vi "SeriellReadFPGA_ECD.vi"   [LabVIEW 2017]
uses:
  <vilib>/rvi/eio/common/nirviEmuTemplateMethod_errors.vi
  <vilib>/rvi/Emulation/niFpgaGetClockAttributes.vi
  <vilib>/rvi/Emulation/niFpgaSctlEmulationGetInTimedLoop.vi
  <vilib>/rvi/Emulation/niFpgaEmulationReportErrorSimple.vi
  GVglobalStopFPGA_ECD.vi
  <vilib>/rvi/DataTransferAndStorage/Container/Common/niFpgaContainerExecOnDevCompGetState.vi
  <vilib>/rvi/Emulation/niFpgaEmulationIsFPGAContextNoSignature.vi
  <vilib>/rvi/errors/niFpgaSetErrorForExecOnDevCompSimple.vi
  <vilib>/rvi/eio/common/nirviEmuReportErrorAndStop.vi
  <vilib>/rvi/DataTransferAndStorage/Container/Common/niFpgaContainerGetUniqueNameForEmu.vi
  <vilib>/rvi/FIFO/Fifo_Resource/nirvififoEmulationSetSize.vi
  <vilib>/rvi/FIFO/Fifo_Resource/nirviFifoEmulationQueueMgr.vi
  <instcachedir>/0/nirviFifoEmulationQueueMgr_E5CAEC123FF24DC58D834DCA3CDAA9B5.lvgen/nirviFifoEmulationQueueMgr_E5CAEC123FF24DC58D834DCA3CDAA9B5_002.vi
  <vilib>/rvi/FIFO/Fifo_Resource/nirvififoEmulationDetermineInputValidOut.vi
  <vilib>/rvi/FIFO/Fifo_Resource/nirvififoEmulationCreateLock.vi
  <vilib>/rvi/Emulation/niFpgaProcessEmulError.vi
  <vilib>/rvi/FIFO/Fifo_Resource/nirvififoEmulationObtainLock.vi
  <vilib>/rvi/FIFO/Fifo_Resource/nirvififoEmulationReleaseLock.vi
  <vilib>/rvi/occurrence/nirviWaitOnOccurrenceBase.vi
  <vilib>/rvi/errors/nirviReportUnexpectedCaseInternalError.vi
  <vilib>/rvi/errors/nirviReportUnexpectedCaseInternalError (U32).vi
  <vilib>/Utility/error.llb/Clear Errors.vi
  <vilib>/rvi/interface/RandomDataEmulation/niFpgaRandomDataHandleErrors.vi
  <vilib>/rvi/Emulation/niFpgaCriticalErrorInLSC.vi
  <vilib>/eio/EIOMethodNode/EIOMethodNode.xnode
  <vilib>/rvi/DataTransferAndStorage/Container/XNode/niFpgaContainer.xnode
  <vilib>/rvi/FIFO/Fifo_Resource/niFpgaFifoEmulationRefIn.vi
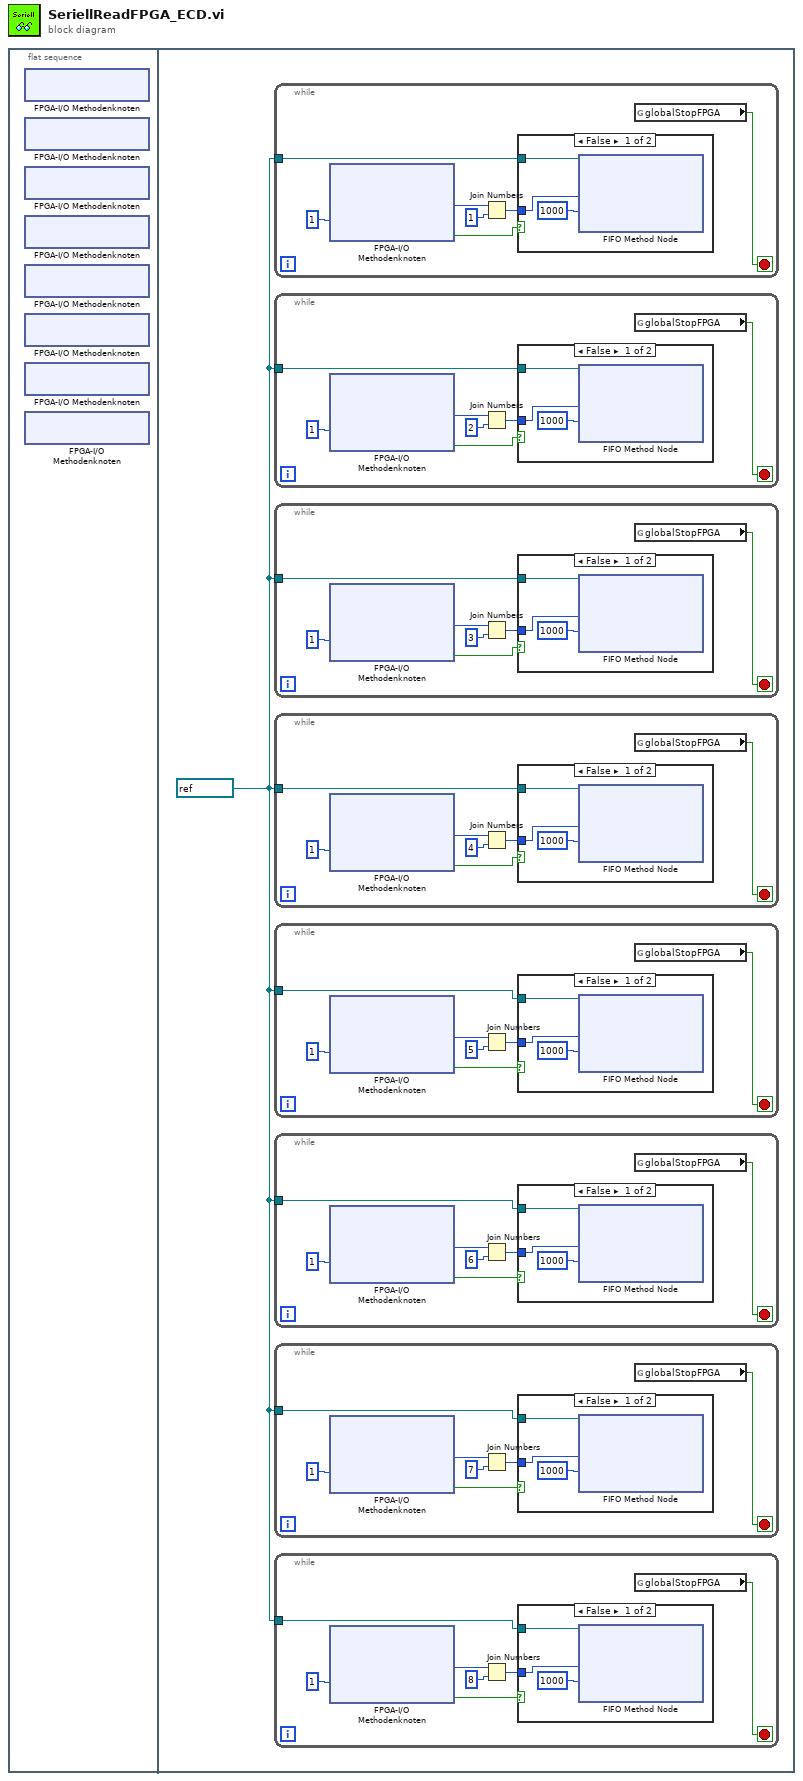
[diagram p0: block diagram]
diagram:
  n1 = flat-sequence {
    frame #0 {
      n2 = xnode "FPGA-I/O Methodenknoten"() -> ()  [unwired: 1 in, 1 out]
      n3 = xnode "FPGA-I/O Methodenknoten"() -> ()  [unwired: 1 in, 1 out]
      n4 = xnode "FPGA-I/O Methodenknoten"() -> ()  [unwired: 1 in, 1 out]
      n5 = xnode "FPGA-I/O Methodenknoten"() -> ()  [unwired: 1 in, 1 out]
      n6 = xnode "FPGA-I/O Methodenknoten"() -> ()  [unwired: 1 in, 1 out]
      n7 = xnode "FPGA-I/O Methodenknoten"() -> ()  [unwired: 1 in, 1 out]
      n8 = xnode "FPGA-I/O Methodenknoten"() -> ()  [unwired: 1 in, 1 out]
      n9 = xnode "FPGA-I/O Methodenknoten"() -> ()  [unwired: 1 in, 1 out]
    }
    frame #1 {
      w1 = refnum<k21> "READ" ("FIFO (Eingang)")
      n10 = while {
        tunnel: w1 -> [w72]
        stop <- w73 stop-if-true
        n11 = xnode "FPGA-I/O Methodenknoten"("Timeout (ms)"=1) -> ("Data"=w78:u8, "Timed Out"=w76:bool)  [unwired: 1 in, 1 out]
        n12 = Join Numbers(hi=w78, lo=u8 1) -> ((hi.lo)=w75:u16)
        n13 = case shown="False" w76 {
          tunnel: w75 -> [w81 _]
          tunnel: w72 -> [w79 _]
          frame False {
            n14 = xnode ("FIFO Method Node")("Element"=w81, "Timeout"=1000, "FIFO (Eingang)"=w79) -> ()  [unwired: 2 out]
          }
          frame True {
          }
        }
        n15 = global read "GVglobalStopFPGA_ECD.vi" "globalStopFPGA"() -> (w73:bool)
      }
      n16 = while {
        tunnel: w1 -> [w62]
        stop <- w63 stop-if-true
        n17 = xnode "FPGA-I/O Methodenknoten"("Timeout (ms)"=1) -> ("Data"=w68:u8, "Timed Out"=w66:bool)  [unwired: 1 in, 1 out]
        n18 = Join Numbers(hi=w68, lo=u8 2) -> ((hi.lo)=w65:u16)
        n19 = case shown="False" w66 {
          tunnel: w65 -> [w71 _]
          tunnel: w62 -> [w69 _]
          frame False {
            n20 = xnode ("FIFO Method Node")("Element"=w71, "Timeout"=1000, "FIFO (Eingang)"=w69) -> ()  [unwired: 2 out]
          }
          frame True {
          }
        }
        n21 = global read "GVglobalStopFPGA_ECD.vi" "globalStopFPGA"() -> (w63:bool)
      }
      n22 = while {
        tunnel: w1 -> [w52]
        stop <- w53 stop-if-true
        n23 = xnode "FPGA-I/O Methodenknoten"("Timeout (ms)"=1) -> ("Data"=w58:u8, "Timed Out"=w56:bool)  [unwired: 1 in, 1 out]
        n24 = Join Numbers(hi=w58, lo=u8 3) -> ((hi.lo)=w55:u16)
        n25 = case shown="False" w56 {
          tunnel: w55 -> [w61 _]
          tunnel: w52 -> [w59 _]
          frame False {
            n26 = xnode ("FIFO Method Node")("Element"=w61, "Timeout"=1000, "FIFO (Eingang)"=w59) -> ()  [unwired: 2 out]
          }
          frame True {
          }
        }
        n27 = global read "GVglobalStopFPGA_ECD.vi" "globalStopFPGA"() -> (w53:bool)
      }
      n28 = while {
        tunnel: w1 -> [w42]
        stop <- w43 stop-if-true
        n29 = xnode "FPGA-I/O Methodenknoten"("Timeout (ms)"=1) -> ("Data"=w48:u8, "Timed Out"=w46:bool)  [unwired: 1 in, 1 out]
        n30 = Join Numbers(hi=w48, lo=u8 4) -> ((hi.lo)=w45:u16)
        n31 = case shown="False" w46 {
          tunnel: w45 -> [w51 _]
          tunnel: w42 -> [w49 _]
          frame False {
            n32 = xnode ("FIFO Method Node")("Element"=w51, "Timeout"=1000, "FIFO (Eingang)"=w49) -> ()  [unwired: 2 out]
          }
          frame True {
          }
        }
        n33 = global read "GVglobalStopFPGA_ECD.vi" "globalStopFPGA"() -> (w43:bool)
      }
      n34 = while {
        tunnel: w1 -> [w32]
        stop <- w33 stop-if-true
        n35 = xnode "FPGA-I/O Methodenknoten"("Timeout (ms)"=1) -> ("Data"=w38:u8, "Timed Out"=w36:bool)  [unwired: 1 in, 1 out]
        n36 = Join Numbers(hi=w38, lo=u8 5) -> ((hi.lo)=w35:u16)
        n37 = case shown="False" w36 {
          tunnel: w35 -> [w41 _]
          tunnel: w32 -> [w39 _]
          frame False {
            n38 = xnode ("FIFO Method Node")("Element"=w41, "Timeout"=1000, "FIFO (Eingang)"=w39) -> ()  [unwired: 2 out]
          }
          frame True {
          }
        }
        n39 = global read "GVglobalStopFPGA_ECD.vi" "globalStopFPGA"() -> (w33:bool)
      }
      n40 = while {
        tunnel: w1 -> [w22]
        stop <- w23 stop-if-true
        n41 = xnode "FPGA-I/O Methodenknoten"("Timeout (ms)"=1) -> ("Data"=w28:u8, "Timed Out"=w26:bool)  [unwired: 1 in, 1 out]
        n42 = Join Numbers(hi=w28, lo=u8 6) -> ((hi.lo)=w25:u16)
        n43 = case shown="False" w26 {
          tunnel: w25 -> [w31 _]
          tunnel: w22 -> [w29 _]
          frame False {
            n44 = xnode ("FIFO Method Node")("Element"=w31, "Timeout"=1000, "FIFO (Eingang)"=w29) -> ()  [unwired: 2 out]
          }
          frame True {
          }
        }
        n45 = global read "GVglobalStopFPGA_ECD.vi" "globalStopFPGA"() -> (w23:bool)
      }
      n46 = while {
        tunnel: w1 -> [w12]
        stop <- w13 stop-if-true
        n47 = xnode "FPGA-I/O Methodenknoten"("Timeout (ms)"=1) -> ("Data"=w18:u8, "Timed Out"=w16:bool)  [unwired: 1 in, 1 out]
        n48 = Join Numbers(hi=w18, lo=u8 7) -> ((hi.lo)=w15:u16)
        n49 = case shown="False" w16 {
          tunnel: w15 -> [w21 _]
          tunnel: w12 -> [w19 _]
          frame False {
            n50 = xnode ("FIFO Method Node")("Element"=w21, "Timeout"=1000, "FIFO (Eingang)"=w19) -> ()  [unwired: 2 out]
          }
          frame True {
          }
        }
        n51 = global read "GVglobalStopFPGA_ECD.vi" "globalStopFPGA"() -> (w13:bool)
      }
      n52 = while {
        tunnel: w1 -> [w2]
        stop <- w3 stop-if-true
        n53 = xnode "FPGA-I/O Methodenknoten"("Timeout (ms)"=1) -> ("Data"=w8:u8, "Timed Out"=w6:bool)  [unwired: 1 in, 1 out]
        n54 = Join Numbers(hi=w8, lo=u8 8) -> ((hi.lo)=w5:u16)
        n55 = case shown="False" w6 {
          tunnel: w5 -> [w11 _]
          tunnel: w2 -> [w9 _]
          frame False {
            n56 = xnode ("FIFO Method Node")("Element"=w11, "Timeout"=1000, "FIFO (Eingang)"=w9) -> ()  [unwired: 2 out]
          }
          frame True {
          }
        }
        n57 = global read "GVglobalStopFPGA_ECD.vi" "globalStopFPGA"() -> (w3:bool)
      }
    }
  }
